vi "VG_OCV70min_P.vi"() -> ()   [LabVIEW 2020]
panel:
  out "OCV70min":dbl
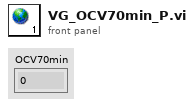
[diagram p1: front panel]
diagram:
